vi "Decimation Page.vi"(8 "error in (no error)":errorcluster, 11 "Node Ptr":T1 format="%.0x") -> (0 "error out":errorcluster)   [LabVIEW 2027, in "Embedded Data Logger System Explorer.lvlib"]
uses:
  Embedded Data Logger System Explorer.lvlib
  <vilib>/NI VeriStand/Custom Device API/Custom Device Item Ref.ctl
  <vilib>/NI VeriStand/Custom Device API/Custom Device API.lvlib
panel:
  in  "Default Decimation":i32=1 min=1
  in  "Header":cluster{"Section Name":string}={"Section Name"="Decimation Channel Settings"}
  out "Description":string
  in  "Name":string
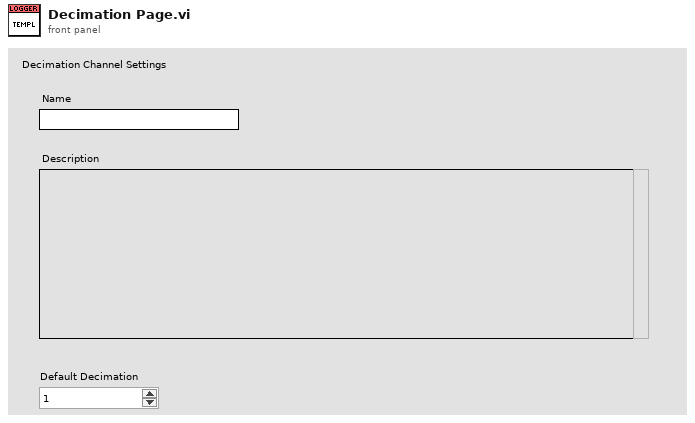
[diagram p1: front panel]
types:
  T1 = typedef "Custom Device API.lvlib/Custom Device Item Ref.ctl" = u64
  T2 = typedef "Custom Device API.lvlib/Custom Device Item Info.ctl" = cluster{"Name":string, "Is Channel":bool, "GUID":string, "Is Waveform":bool}
  T3 = typedef "Custom Device API.lvlib/Custom Device Channel.ctl" = cluster{"Type":T4, "Units":string, "Default Value":dbl, "Faultable":bool, "Scalable":bool}
  T4 = typedef "Custom Device API.lvlib/Custom Device Channel Type.ctl" = enum16{"Input", "Output"}
  T5 = typedef "Custom Device API.lvlib/Custom Device Commands.ctl" = enum16{"Default", "Item renamed", "Shutdown", "Dynamic button pressed"}
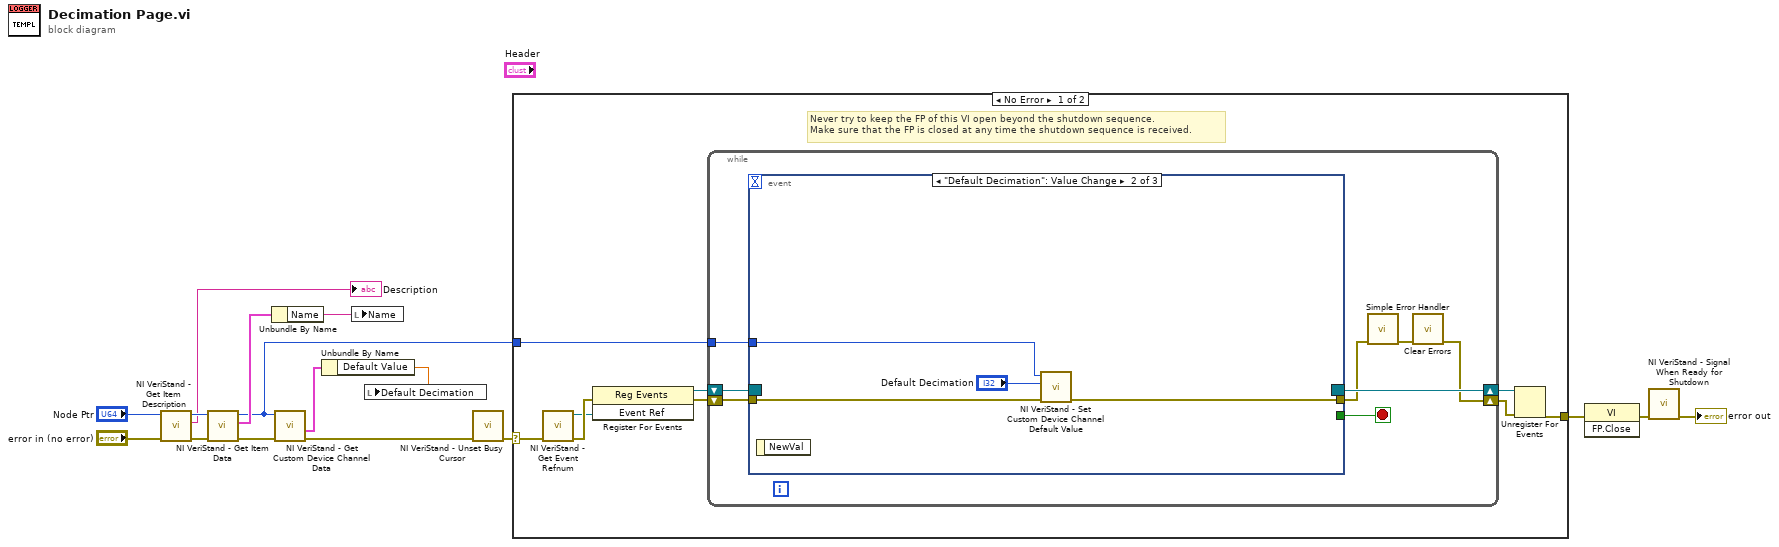
[diagram p0: block diagram]
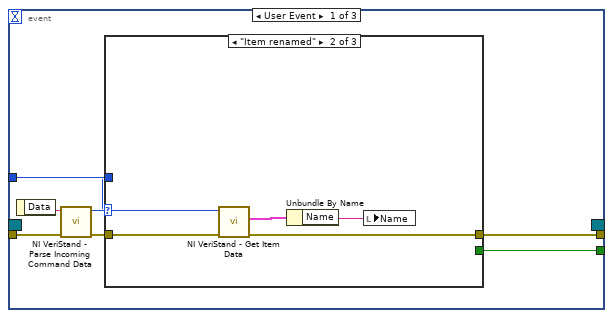
[diagram p2: hidden frame]
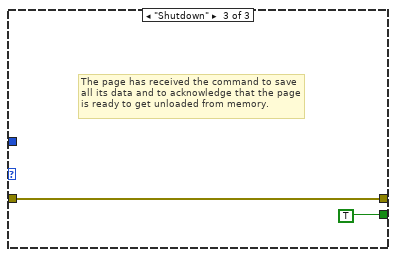
[diagram p4: hidden frame]
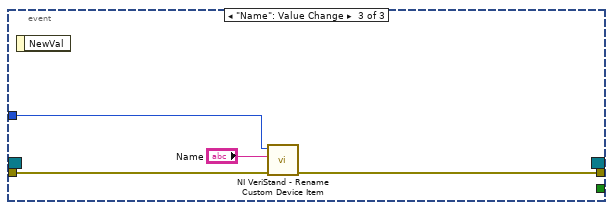
[diagram p5: hidden frame]
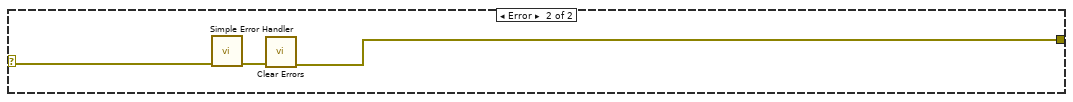
[diagram p6: hidden frame]
diagram:
  n1 = call <vilib>:"NI VeriStand - Get Item Description.vi"("error in (no error)"="error in (no error)", "Item Ref in"="Node Ptr") -> ("error out"=w9:errorcluster, "Description"=→"Description":string, "Item Ref out"=w10:T1)  [unwired: 7 out]
  n2 = call <vilib>:"NI VeriStand - Get Item Data.vi"("error in (no error)"=w9, "Item Ref in"=w10) -> ("error out"=w6:errorcluster, "Item Info"=w8:T2, "Item Ref out"=w5:T1)  [unwired: 7 out]
  n3 = Unbundle By Name(w8) -> ("Name"=w7:string)
  n4 = call <vilib>:"NI VeriStand - Get Custom Device Channel Data.vi"("error in (no error)"=w6, "Channel Ref in"=w5) -> ("error out"=w4:errorcluster, "Channel"=w3:T3)  [unwired: 8 out]
  n5 = Unbundle By Name(w3) -> ("Default Value"=w2:dbl)
  n6 = local write "Name"(w7) -> ()
  n7 = local write "Default Decimation"(w2) -> ()
  n8 = call <vilib>:"NI VeriStand - Unset Busy Cursor.vi"("error in (no error)"=w4) -> ("error out"=w12:errorcluster)  [unwired: 10 out]
  n9 = case shown="No Error" w12 {
    selector: w12 -> [w17 w59]
    tunnel: [w22 w57] -> w16
    tunnel: w5 -> [w18 _]
    frame No Error {
      # "Never try to keep the FP of this VI open beyond the shutdown sequence.\nMake sure that the FP is closed at any time the shutdown sequence is received."
      n10 = call <vilib>:"NI VeriStand - Get Event Refnum.vi"("error in (no error)"=w17) -> ("error out"=w25:errorcluster, "Event Ref"=w21:refnum<user-event>)  [unwired: 9 out]
      n11 = register-events(error in=w25, w21) -> (reference out=w19:refnum<event-registration>, error out=w20:errorcluster)  [unwired: 1 in]
      n12 = while {
        tunnel: w18 -> [w29]
        shift-right: [w26] -> w23
        shift-left: w20 -> [w32]
        shift-right: [w33] -> w24
        shift-left: w19 -> [w31]
        stop <- w30 stop-if-true
        n13 = event shown="[1] \"Default Decimation\": Value Change" {
          selector: w31 -> [_ _ _]
          dyn-events: [_ _ _] -> w33
          timeout: _ -> [_ _ _]
          tunnel: w32 -> [w40 w52 w56]
          tunnel: [w36 _ _] -> w30
          tunnel: [w35 w50 w55] -> w28
          tunnel: w29 -> [w34 w51 w54]
          event User Event {
            n14 = event-data() -> ("Data"=w39:string)  [unwired: 1 out]
            n15 = call <vilib>:"NI VeriStand - Parse Incoming Command Data.vi"("error in (no error)"=w40, "Incoming data"=w39) -> ("error out"=w38:errorcluster, "Action"=w37:T5)  [unwired: 8 out]
            n16 = case shown="\"Item renamed\"" w37 {
              tunnel: w38 -> [w41 w46 w47]
              tunnel: [_ _ TRUE] -> w36
              tunnel: [w41 w43 w47] -> w35
              tunnel: w34 -> [_ w45 _]
              frame "Default", Default {
              }
              frame "Item renamed" {
                n17 = call <vilib>:"NI VeriStand - Get Item Data.vi"("error in (no error)"=w46, "Item Ref in"=w45) -> ("error out"=w43:errorcluster, "Item Info"=w44:T2)  [unwired: 8 out]
                n18 = Unbundle By Name(w44) -> ("Name"=w42:string)
                n19 = local write "Name"(w42) -> ()
              }
              frame "Shutdown" {
                # "The page has received the command to save all its data and to acknowledge that the page is ready to get unloaded from memory."
              }
            }
          }
          event "Default Decimation": Value Change {
            n20 = event-data() -> ()  [unwired: 2 out]
            n21 = call <vilib>:"NI VeriStand - Set Custom Device Channel Default Value.vi"("error in (no error)"=w52, "Default Value"="Default Decimation", "Channel Ref in"=w51) -> ("error out"=w50:errorcluster)  [unwired: 8 out]
          }
          event "Name": Value Change {
            n22 = event-data() -> ()  [unwired: 2 out]
            n23 = call <vilib>:"NI VeriStand - Rename Custom Device Item.vi"("error in (no error)"=w56, "New Name"="Name", "Item Ref in"=w54) -> ("error out"=w55:errorcluster)  [unwired: 1 in, 7 out]
          }
        }
        n24 = call <vilib>:"Simple Error Handler.vi"("error in (no error)"=w28) -> ("error out"=w27:errorcluster)  [unwired: 1 in, 7 out]
        n25 = call <vilib>:"Clear Errors.vi"("error in (no error)"=w27) -> ("error out"=w26:errorcluster)  [unwired: 1 in, 5 out]
      }
      n26 = Unregister For Events(event registration refnum=w24, error in=w23) -> (error out=w22:errorcluster)
    }
    frame Error {
      n27 = call <vilib>:"Simple Error Handler.vi"("error in (no error)"=w59) -> ("error out"=w58:errorcluster)  [unwired: 1 in, 7 out]
      n28 = call <vilib>:"Clear Errors.vi"("error in (no error)"=w58) -> ("error out"=w57:errorcluster)  [unwired: 1 in, 5 out]
    }
  }
  n29 = invoke class="VI" method="FP.Close"(error in=w16) -> (error out=w15:errorcluster)  [unwired: 2 in, 2 out]
  n30 = call <vilib>:"NI VeriStand - Signal When Ready for Shutdown.vi"("error in (no error)"=w15) -> ("error out"=→"error out":errorcluster)  [unwired: 10 out]
